vi "Stop.vi"(8 "error in (no error)":errorcluster, 11 "JQMHCore in":refnum<class "JQMHModule.lvclass">) -> (0 "error out":errorcluster, 3 "JQMHCore out":refnum<class "JQMHModule.lvclass">)   [LabVIEW 2024, in "JQMHModule.lvclass"]
uses:
  JQMHModule.lvclass
  JQMHModule.lvclass/JQMHModule.ctl
  Message Queue_class/Delacor_lib_QMH_Message Queue.lvclass/Delacor_lib_QMH_Message Queue.ctl
  <vilib>/Delacor/Delacor QMH/Libraries/Message Queue_class/Delacor_lib_QMH_Enqueue Message (Single).vi
  Message Queue_class/Delacor_lib_QMH_Message Queue.lvclass
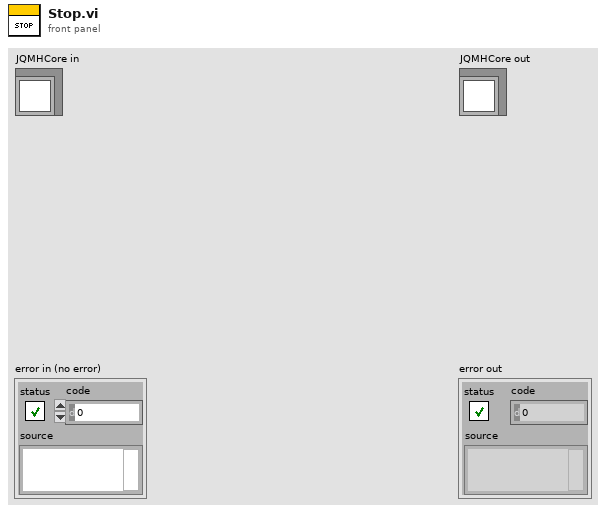
[diagram p1: front panel]
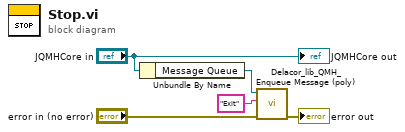
[diagram p0: block diagram]
diagram:
  n1 = Unbundle By Name("JQMHCore in") -> ("Message Queue"=w4:refnum<class "Delacor_lib_QMH_Message Queue.lvclass">)
  n2 = call-poly <vilib>:"Delacor_lib_QMH_Enqueue Message (poly).vi"("error in"="error in (no error)", "Message"="Exit", "Message Queue in"=w4) -> ("error out"=→"error out":errorcluster)  [unwired: 7 in, 1 out]
  "JQMHCore out" <- "JQMHCore in"
